vi "Output_opt.vi"(0 "Activation Function":enum32{"Sigmoid", "RELU", "Tanh", "Leaky RELU"}(ring), 1 "Activation l-1":dbl[](array[numeric]), 2 "Weights":dbl[](array[numeric]), 3 "Biases":dbl, 5 "Activation":dbl, 7 "Net Output":dbl, 9 "Target":dbl, 13 "Adam Data In":T1) -> (4 "Delta":dbl, 6 "Updated Weights":dbl[](array[numeric]), 8 "Updated Biases":dbl, 14 "Adam Data Out":T1)   [LabVIEW 2018]
uses:
  Adam_data.ctl
  Globals.vi
  Optimizer.vi
  Iteration Counter.vi
panel:
  out "Grad. w":dbl[](array[numeric])
  out "Grad. b":dbl
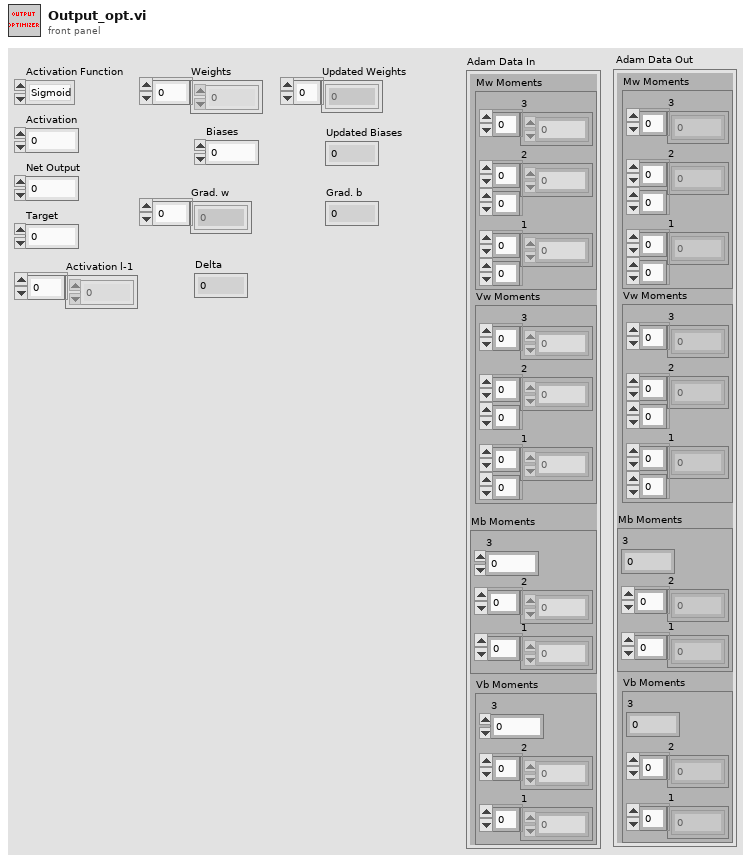
[diagram p1: front panel]
types:
  T1 = typedef "Adam_data.ctl" = cluster{"Mw Moments":cluster{"3 ":dbl[], "2":dbl[][], "1":dbl[][]}, "Vw Moments":cluster{"3":dbl[], "2":dbl[][], "1":dbl[][]}, "Mb Moments":cluster{"3":dbl, "2":dbl[], "1":dbl[]}, "Vb Moments":cluster{"3":dbl, "2":dbl[], "1":dbl[]}}
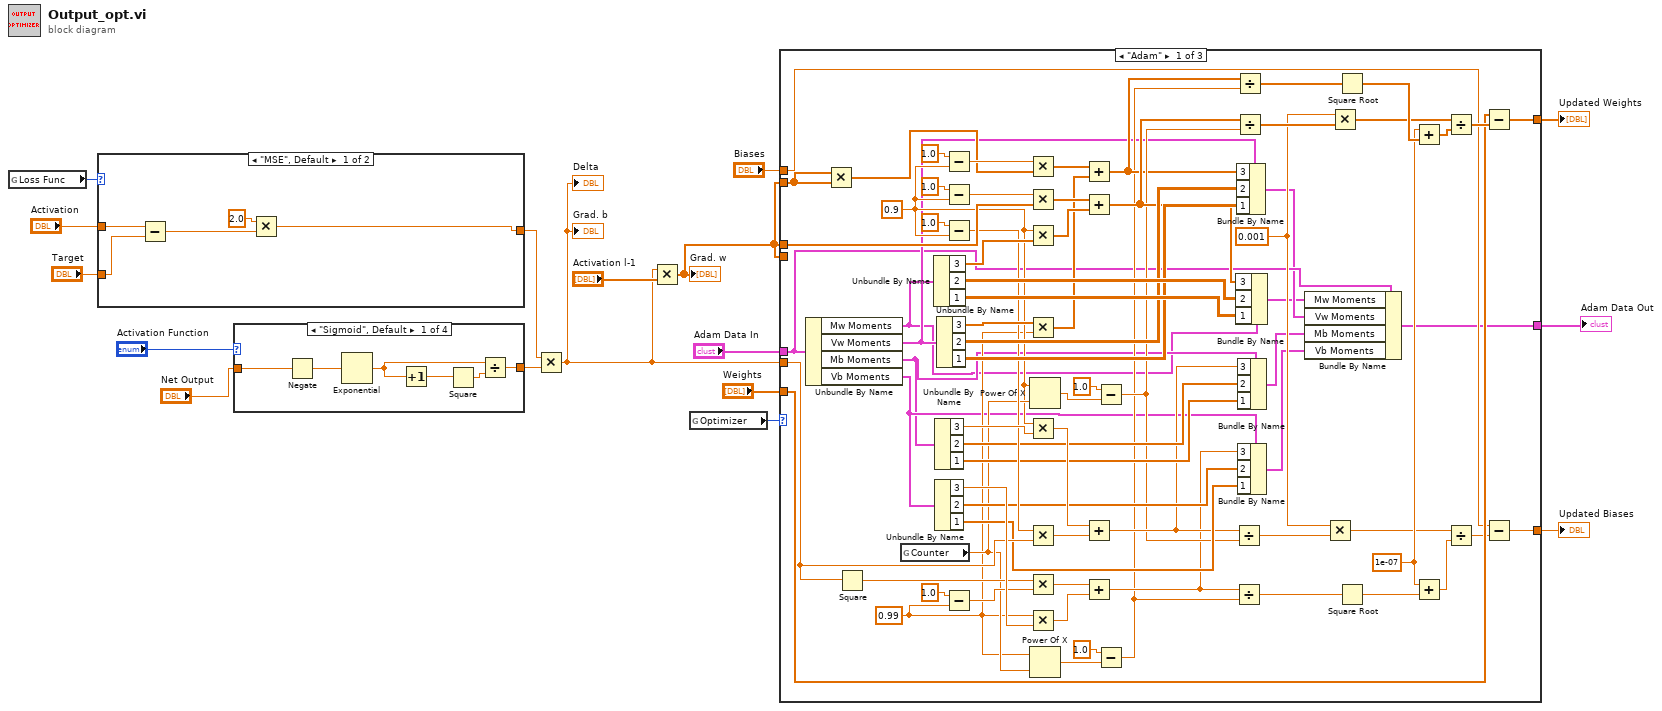
[diagram p0: block diagram]
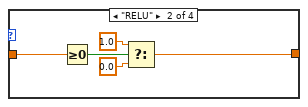
[diagram p4: hidden frame]
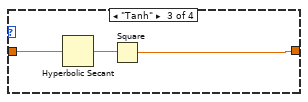
[diagram p5: hidden frame]
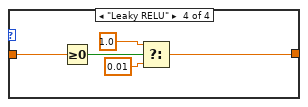
[diagram p6: hidden frame]
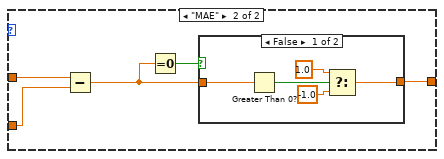
[diagram p7: hidden frame]
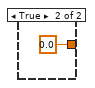
[diagram p8: hidden frame]
diagram:
  n1 = global read "Globals.vi" "Loss Func"() -> (w17:enum16{"MSE", "MAE"})
  n2 = case shown="\"MSE\", Default" w17 {
    tunnel: "Activation" -> [w21 w26]
    tunnel: "Target" -> [w20 w27]
    tunnel: [w18 w24] -> w13
    frame "MSE", Default {
      n3 = Subtract(x=w21, y=w20) -> (x-y=w19:dbl)
      n4 = Multiply(x=2.0, y=w19) -> (x*y=w18:dbl)
    }
    frame "MAE" {
      n5 = Subtract(x=w26, y=w27) -> (x-y=w23:dbl)
      n6 = Equal To 0?(x=w23) -> (x = 0?=w25:bool)
      n7 = case shown="False" w25 {
        tunnel: [w28 0.0] -> w24
        tunnel: w23 -> [w32 _]
        frame False {
          n8 = Greater Than 0?(x=w32) -> (x > 0?=w31:bool)
          n9 = Select(t=1.0, s=w31, f=-1.0) -> (s? t:f=w28:dbl)
        }
        frame True {
        }
      }
    }
  }
  n10 = case shown="\"Sigmoid\", Default" "Activation Function" {
    tunnel: "Net Output" -> [w35 w43 w46 w50]
    tunnel: [w34 w44 w45 w49] -> w12
    frame "Sigmoid", Default {
      n11 = Negate(x=w35) -> (-x=w39:dbl)
      n12 = Exponential(1:w39) -> (0:w36:dbl)
      n13 = Increment(x=w36) -> (x+1=w38:dbl)
      n14 = Square(x=w38) -> (x^2=w37:dbl)
      n15 = Divide(x=w36, y=w37) -> (x/y=w34:dbl)
    }
    frame "RELU" {
      n16 = Greater Or Equal To 0?(x=w43) -> (x >= 0?=w40:bool)
      n17 = Select(t=1.0, s=w40, f=0.0) -> (s? t:f=w44:dbl)
    }
    frame "Tanh" {
      n18 = Hyperbolic Secant(1:w46) -> (0:w47:dbl)
      n19 = Square(x=w47) -> (x^2=w45:dbl)
    }
    frame "Leaky RELU" {
      n20 = Greater Or Equal To 0?(x=w50) -> (x >= 0?=w48:bool)
      n21 = Select(t=1.0, s=w48, f=0.01) -> (s? t:f=w49:dbl)
    }
  }
  n22 = Multiply(x=w13, y=w12) -> (x*y=w7:dbl)
  "Delta" <- w7
  "Grad. b" <- w7
  n23 = Multiply(x=w7, y="Activation l-1") -> (x*y=w8:dbl[])
  "Grad. w" <- w8
  n24 = global read "Optimizer.vi" "Optimizer"() -> (w9:enum16{"Adagrad", "Adadelta", "Adam"})
  n25 = case shown="\"Adam\"" w9 {
    tunnel: w8 -> [_ _ _]
    tunnel: w8 -> [w122 _ _]
    tunnel: w8 -> [w115 _ _]
    tunnel: w7 -> [w100 _ _]
    tunnel: "Weights" -> [w74 w129 w132]
    tunnel: [w73 w129 w132] -> w5
    tunnel: "Biases" -> [w65 w128 w131]
    tunnel: [w63 w128 w131] -> w3
    tunnel: "Adam Data In" -> [w58 w127 w130]
    tunnel: [w53 w127 w130] -> w1
    frame "Adam" {
      w70 = 1e-07
      w69 = 0.001
      w91 = 0.99
      w92 = 0.9
      n26 = Unbundle By Name(w58) -> ("Mw Moments"=w59:cluster{"3 ":dbl[], "2":dbl[][], "1":dbl[][]}, "Vw Moments"=w60:cluster{"3":dbl[], "2":dbl[][], "1":dbl[][]}, "Mb Moments"=w61:cluster{"3":dbl, "2":dbl[], "1":dbl[]}, "Vb Moments"=w62:cluster{"3":dbl, "2":dbl[], "1":dbl[]})
      n27 = Multiply(x=w115, y=w115) -> (x*y=w114:dbl[])
      n28 = Square(x=w100) -> (x^2=w98:dbl)
      n29 = global read "Iteration Counter.vi" "Counter"() -> (w93:dbl)
      n30 = Unbundle By Name(w59) -> ("3"=w126:dbl[], "2"=w120:dbl[][], "1"=w119:dbl[][])
      n31 = Unbundle By Name(w61) -> ("3"=w109:dbl, "2"=w104:dbl[], "1"=w103:dbl[])
      n32 = Unbundle By Name(w62) -> ("3"=w102:dbl, "2"=w95:dbl[], "1"=w94:dbl[])
      n33 = Unbundle By Name(w60) -> ("3"=w118:dbl[], "2"=w111:dbl[][], "1"=w110:dbl[][])
      n34 = Subtract(x=1.0, y=w92) -> (x-y=w116:dbl)
      n35 = Subtract(x=1.0, y=w92) -> (x-y=w123:dbl)
      n36 = Subtract(x=1.0, y=w92) -> (x-y=w107:dbl)
      n37 = Subtract(x=1.0, y=w91) -> (x-y=w99:dbl)
      n38 = Multiply(x=w116, y=w114) -> (x*y=w112:dbl[])
      n39 = Multiply(x=w123, y=w122) -> (x*y=w121:dbl[])
      n40 = Multiply(x=w92, y=w126) -> (x*y=w124:dbl[])
      n41 = Multiply(x=w118, y=w91) -> (x*y=w113:dbl[])
      n42 = Multiply(x=w92, y=w109) -> (x*y=w105:dbl)
      n43 = Multiply(x=w107, y=w100) -> (x*y=w106:dbl)
      n44 = Multiply(x=w98, y=w99) -> (x*y=w97:dbl)
      n45 = Multiply(x=w91, y=w102) -> (x*y=w96:dbl)
      n46 = Power Of X(1:w93, 2:w92) -> (0:w89:dbl)
      n47 = Power Of X(1:w93, 2:w91) -> (0:w87:dbl)
      n48 = Add(x=w112, y=w113) -> (x+y=w83:dbl[])
      n49 = Add(x=w121, y=w124) -> (x+y=w86:dbl[])
      n50 = Add(x=w105, y=w106) -> (x+y=w85:dbl)
      n51 = Add(x=w97, y=w96) -> (x+y=w82:dbl)
      n52 = Subtract(x=1.0, y=w89) -> (x-y=w84:dbl)
      n53 = Subtract(x=1.0, y=w87) -> (x-y=w81:dbl)
      n54 = Divide(x=w85, y=w84) -> (x/y=w68:dbl)
      n55 = Divide(x=w82, y=w81) -> (x/y=w72:dbl)
      n56 = Divide(x=w83, y=w81) -> (x/y=w80:dbl[])
      n57 = Divide(x=w86, y=w84) -> (x/y=w78:dbl[])
      n58 = Bundle By Name(cluster=w59, "3"=w86, "2"=w120, "1"=w119) -> (w54:cluster{"3 ":dbl[], "2":dbl[][], "1":dbl[][]})
      n59 = Bundle By Name(cluster=w60, "3"=w83, "2"=w111, "1"=w110) -> (w55:cluster{"3":dbl[], "2":dbl[][], "1":dbl[][]})
      n60 = Bundle By Name(cluster=w61, "3"=w85, "2"=w104, "1"=w103) -> (w56:cluster{"3":dbl, "2":dbl[], "1":dbl[]})
      n61 = Bundle By Name(cluster=w62, "3"=w82, "2"=w95, "1"=w94) -> (w57:cluster{"3":dbl, "2":dbl[], "1":dbl[]})
      n62 = Bundle By Name(cluster=w58, "Mw Moments"=w54, "Vw Moments"=w55, "Mb Moments"=w56, "Vb Moments"=w57) -> (w53:T1)
      n63 = Multiply(x=w69, y=w68) -> (x*y=w67:dbl)
      n64 = Multiply(x=w69, y=w78) -> (x*y=w77:dbl[])
      n65 = Square Root(x=w80) -> (sqrt(x)=w79:dbl[])
      n66 = Square Root(x=w72) -> (sqrt(x)=w71:dbl)
      n67 = Add(x=w70, y=w79) -> (x+y=w76:dbl[])
      n68 = Add(x=w70, y=w71) -> (x+y=w66:dbl)
      n69 = Divide(x=w77, y=w76) -> (x/y=w75:dbl[])
      n70 = Divide(x=w67, y=w66) -> (x/y=w64:dbl)
      n71 = Subtract(x=w74, y=w75) -> (x-y=w73:dbl[])
      n72 = Subtract(x=w65, y=w64) -> (x-y=w63:dbl)
    }
    frame "Adadelta" {
    }
    frame "Adagrad" {
    }
  }
  "Updated Weights" <- w5
  "Updated Biases" <- w3
  "Adam Data Out" <- w1
